vi "Write DIO Lines.vi"(8 "error in (no error)":errorcluster, 10 "DIO Lines":string[](array[string]), 11 "RIO Target Configuration in":refnum<class "RIO Target Configuration.lvclass">) -> (0 "error out":errorcluster, 3 "RIO Target Configuration out":refnum<class "RIO Target Configuration.lvclass">)   [LabVIEW 2014, in "RIO Target Configuration.lvclass"]
uses:
  RIO Target Configuration.lvclass
  <vilib>/NI/Configuration Framework/serializable configuration/NISE_CEF_serializable configuration.lvclass
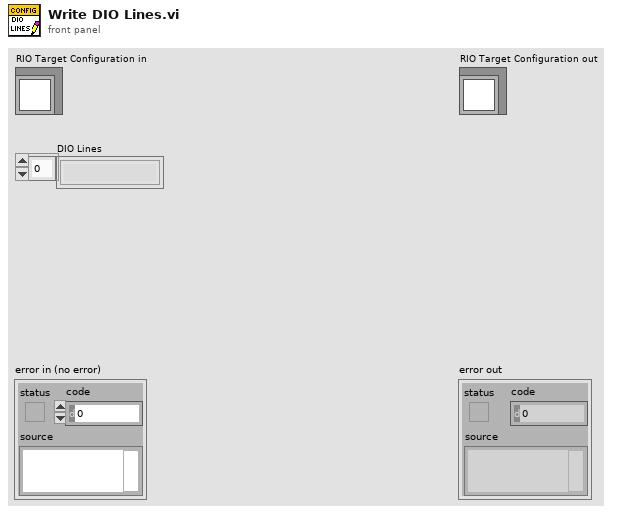
[diagram p1: front panel]
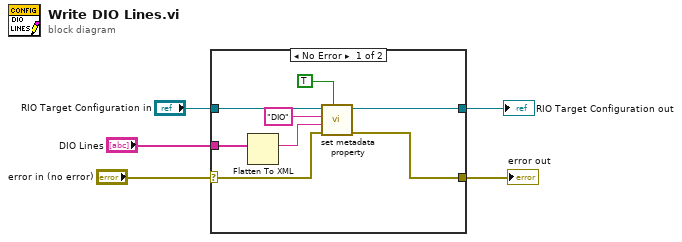
[diagram p0: block diagram]
diagram:
  n1 = case shown="No Error" "error in (no error)" {
    selector: "error in (no error)" -> [w8 w15]
    tunnel: [w10 w15] -> w2
    tunnel: [w12 w14] -> w1
    tunnel: "RIO Target Configuration in" -> [w9 w14]
    tunnel: "DIO Lines" -> [w7 _]
    frame No Error {
      n2 = Flatten To XML(anything=w7) -> (xml string=w6:string)
      n3 = call <vilib>:"set metadata property.vi"("overwrite?"=TRUE, "error in"=w8, "value"=w6, "key"="DIO", "configuration in"=w9) -> ("error out"=w10:errorcluster, "configuration out"=w12:refnum<class "RIO Target Configuration.lvclass">)  [unwired: 5 in]
    }
    frame Error {
    }
  }
  "error out" <- w2
  "RIO Target Configuration out" <- w1
